vi "CODCr固定站质控流程 (子VI).vi"(9 "CODCr量程切换":enum32{"H", "L", "AUTO"}(ring)=enum."AUTO", 10 "CODCr":bool) -> (3 "布尔":bool)   [LabVIEW 2016, in "质控单元.lvlib"]
panel:
  out "参数 out":T1
  out "CODCr中断报警":bool
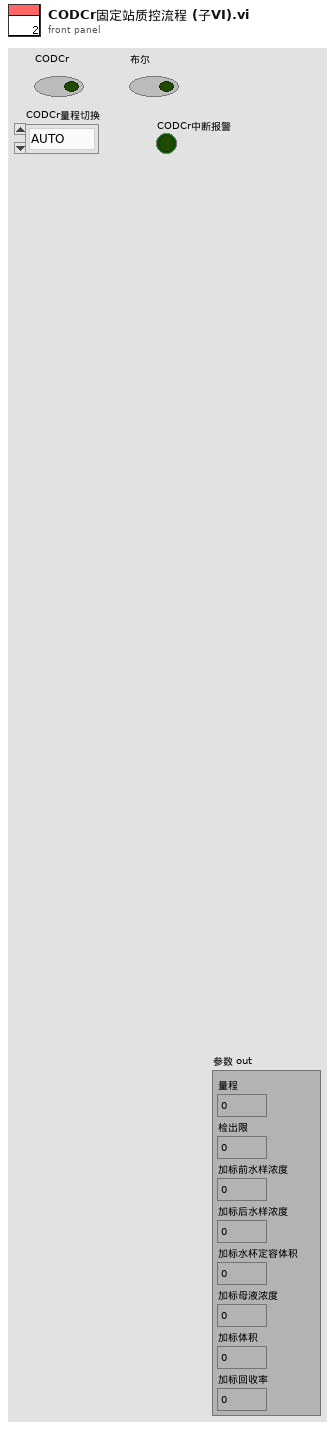
[diagram p1: front panel]
types:
  T1 = cluster{"量程":dbl, "检出限":dbl, "加标前水样浓度":dbl, "加标后水样浓度":dbl, "加标水杯定容体积":dbl, "加标母液浓度":dbl, "加标体积":dbl, "加标回收率":dbl}
  T2 = enum16{"待机", "启动水样测量", "水样测量中", "启动加标", "启动加标回收", "加标回收测量中", "结束"}
  T3 = cluster{"测量模式":enum16{"水样测量", "标样核查", "零点核查", "跨度核查", "空白测试", "加标回收", "平行样", "校零", "校标"}}
  T4 = enum16{"空闲", "水样测试", "标样核查", "零点核查", "跨度核查", "空白测试", "平行样测试", "加标回收", "空白校准", "标样校准", "初始化（清洗）"}
  T5 = cluster{"系统时间":timestamp, "工作状态":enum16{"空闲", "水样测试", "标样核查", "零点核查", "跨度核查", "空白测试", "平行样测试", "加标回收", "空白校准", "标样校准", "初始化（清洗）"}, "测量模式":enum16{"待机", "连续模式", "周期模式", "定点模式", "受控模式", "手动模式"}, "告警代码":enum16{"无告警", "缺试剂告警", "缺水样告警", "缺蒸馏水告警", "缺标液告警", "仪表漏液告警", "标定异常告警", "超量程告警", "加热异常", "低试剂预警", "超上限告警", "超下限告警", "仪表内部其他异常", "滴定异常告警", "电极异常告警", "量程切换告警", "参数设置告警", "PH电极电位异常", "电导率电极异常", "浊度光度异常", "溶解氧电极异常", "溶解氧光强异常", "温度异常告警", "PH异常告警", "溶解氧异常告警", "电导率异常告警", "浊度异常告警", "叶绿素异常告警", "藻密度异常告警", "蓝绿藻异常告警", "ORP异常告警", "氨氮异常告警", "清洁刷异常告警", "SD卡异常告警", "蓝牙异常告警", "Wifi异常告警", "流程异常告警"}, "故障代码":enum16{"无故障", "电机故障", "温度故障", "通讯故障", "滴定故障"}, "日志代码":u16, "软件版本":u16, "F0":sgl, "F1":sgl, "F2":sgl, "F3":sgl, "T":sgl, "H":sgl, "id":u16, "flowid":u16, "量程":u16, "总磷控温温度1":sgl, "营养盐控温温度2":sgl, "ADC":sgl}
  T6 = cluster{"因子编码":u32, "单位":u16, "标样参考值":sgl, "水样数据时间":timestamp, "水样实测值":sgl, "水样数据标识":string, "标样数据时间":timestamp, "标样实测值":sgl, "标样数据标识":string, "空白数据时间":timestamp, "空白实测值":sgl, "空白数据标识":string, "零点核查数据时间":timestamp, "零点核查实测值":sgl, "零点核查数据标识":string, "跨度核查数据时间":timestamp, "跨度核查实测值":sgl, "跨度核查数据标识":string, "加标回收数据时间":timestamp, "加标回收实测值":sgl, "加标回收数据标识":string, "平行样数据时间":timestamp, "平行样实测值":sgl, "平行样数据标识":string}
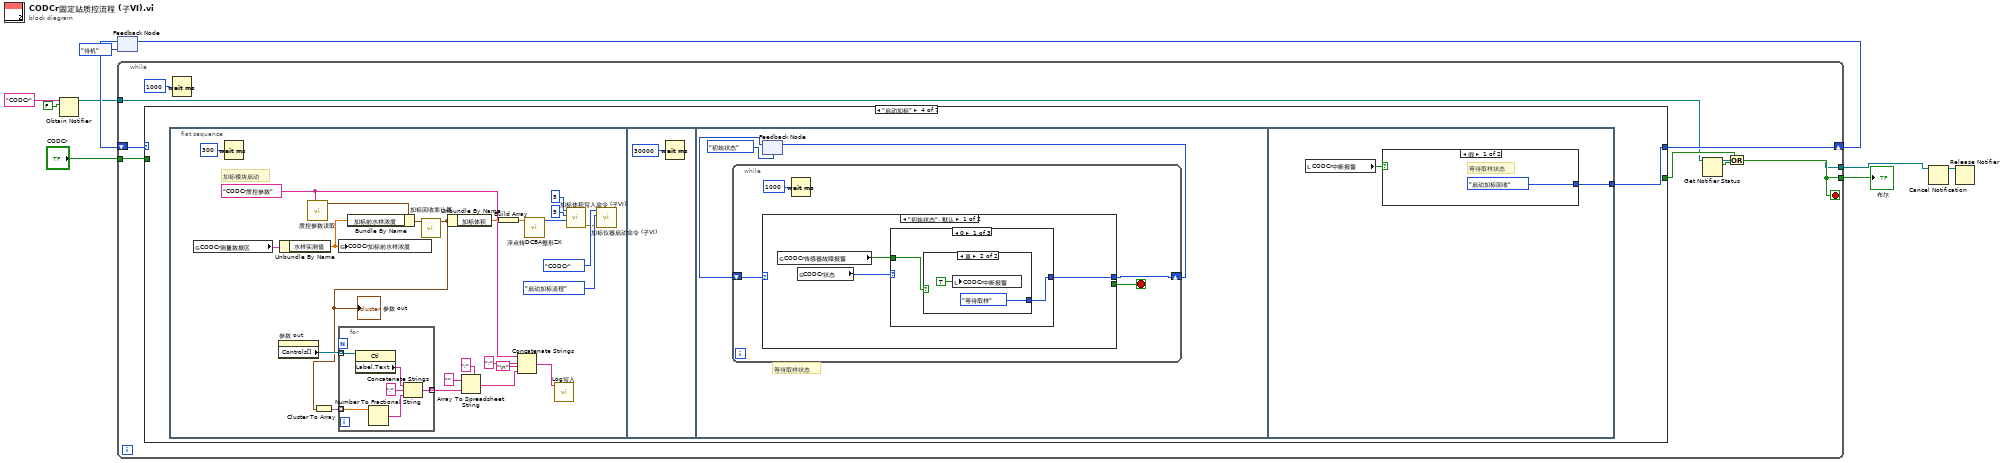
[diagram p0: block diagram]
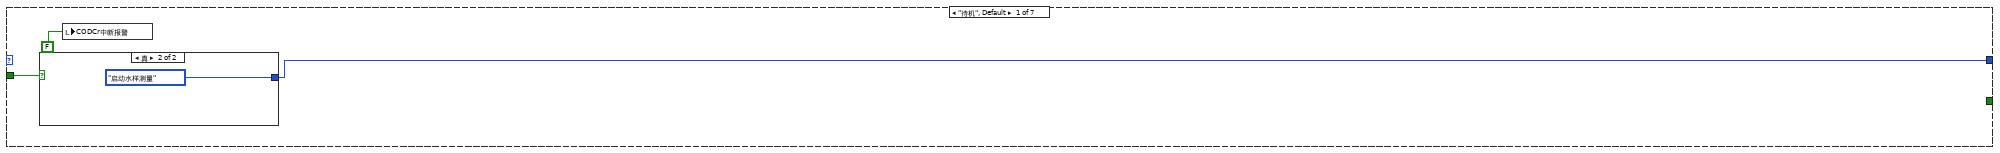
[diagram p2: hidden frame]
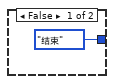
[diagram p3: hidden frame]
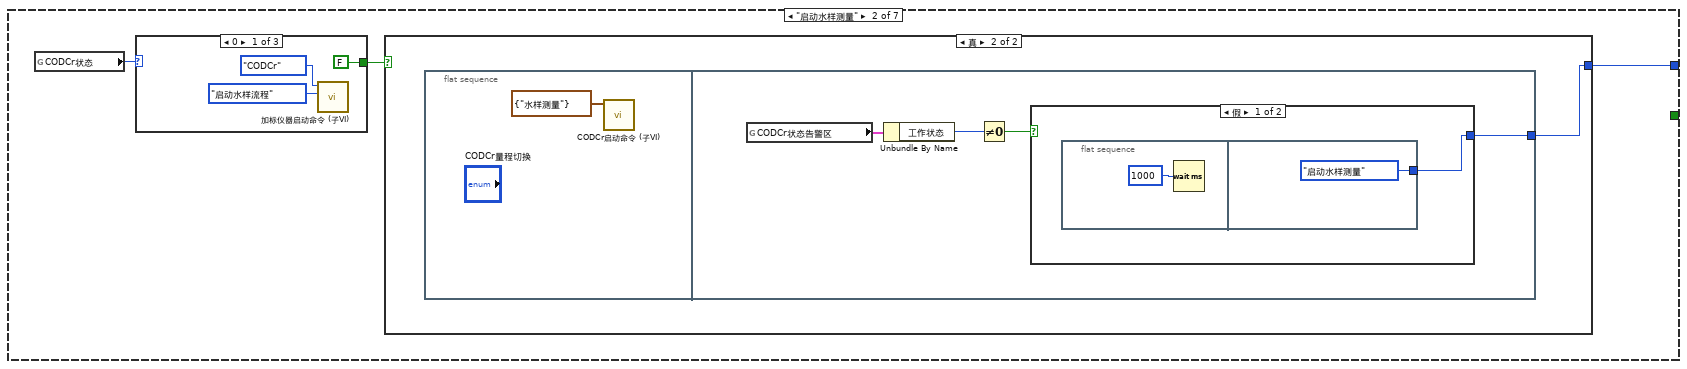
[diagram p4: hidden frame]
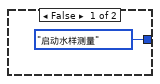
[diagram p5: hidden frame]
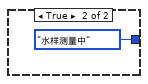
[diagram p6: hidden frame]
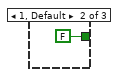
[diagram p7: hidden frame]
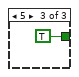
[diagram p8: hidden frame]
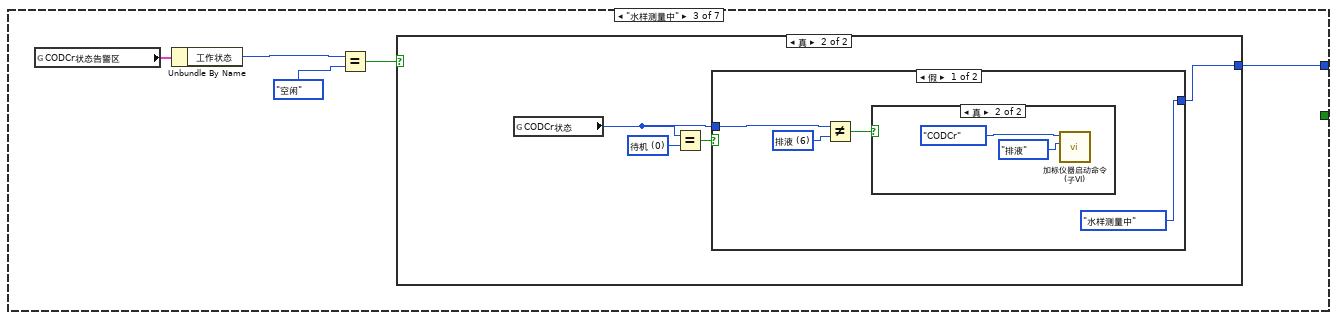
[diagram p9: hidden frame]
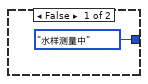
[diagram p10: hidden frame]
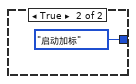
[diagram p12: hidden frame]
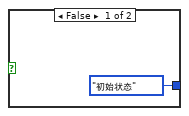
[diagram p13: hidden frame]
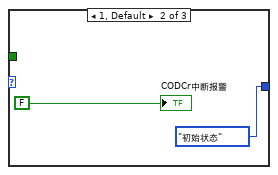
[diagram p14: hidden frame]
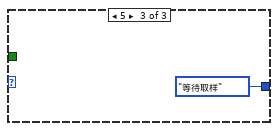
[diagram p15: hidden frame]
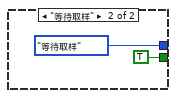
[diagram p16: hidden frame]
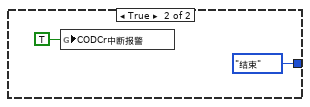
[diagram p17: hidden frame]
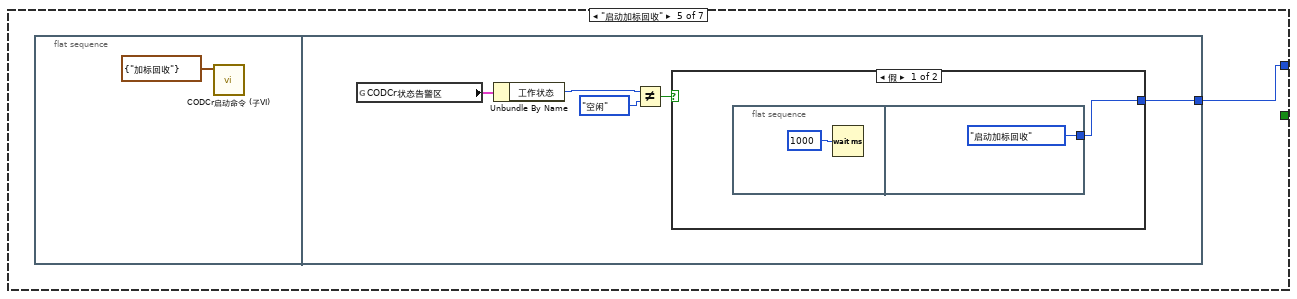
[diagram p18: hidden frame]
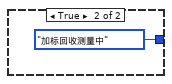
[diagram p19: hidden frame]
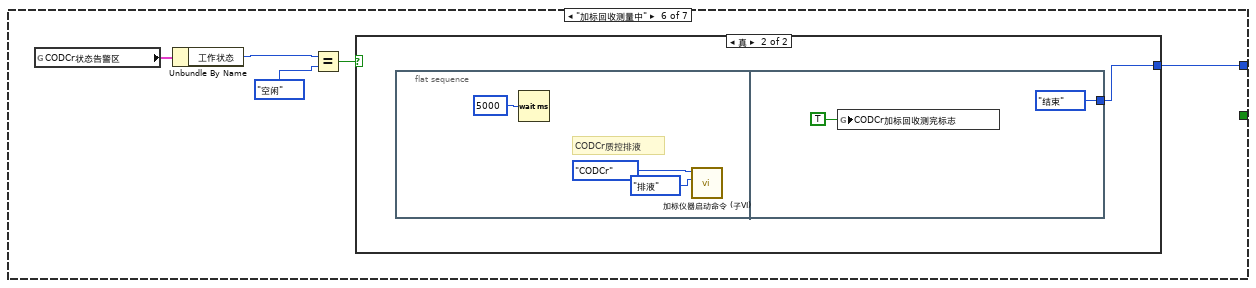
[diagram p20: hidden frame]
diagram:
  n1 = Obtain Notifier(name (unnamed)="CODCr" ("名称（未命名）"), notification data type=FALSE) -> (notifier out=w3:refnum<notifier>)  [unwired: 2 in, 2 out]
  n2 = feedback #1(T2."待机") -> (w6:T2)
  n3 = while {
    tunnel: "CODCr" -> [w19]
    tunnel: [w13] -> w8
    shift-right: [w18] -> w9
    shift-left: w6 -> [w17]
    tunnel: w3 -> [w12]
    tunnel: [w11] -> w1
    stop <- w13 stop-if-true
    n4 = case shown="\"启动加标\"" w17 {
      tunnel: [w22 w27 w48 w61 w118 w133 T2."结束"] -> w18
      tunnel: [_ _ _ _ _ _ TRUE] -> w14
      tunnel: w19 -> [w21 _ _ _ _ _ _]
      frame "待机", Default {
        n5 = case shown="真" w21 {
          tunnel: [T2."结束" T2."启动水样测量"] -> w22
          frame False {
          }
          frame True {
          }
        }
        n6 = local write "CODCr中断报警"(FALSE ("CODMn中断报警")) -> ()
      }
      frame "启动水样测量" {
        n7 = global read "加标回收状态全局变量.vi" "CODCr状态"() -> (w26:u16)
        n8 = case shown="0" w26 {
          tunnel: [FALSE ("s") FALSE ("s") TRUE ("s")] -> w25
          frame 0 {
            n9 = call "加标仪器启动命令 (子VI).vi"("启动命令"=enum16{"启动水样流程", "启动加标流程", "排液", "停止"}."启动水样流程", "仪器"=enum16{"", "氨氮", "总磷", "总氮", "CODMn", "CODCr"}."CODCr") -> ()  [unwired: 9 in, 1 out]
          }
          frame 1, Default {
          }
          frame 5 {
          }
        }
        n10 = case shown="真" w25 {
          tunnel: [T2."启动水样测量" w29] -> w27
          frame False {
          }
          frame True {
            n11 = flat-sequence {
              tunnel: [w34] -> w29
              frame #0 {
                n12 = call "CODCr启动命令 (子VI).vi"("启动测量模式"=T3 {"测量模式"=enum."水样测量"}) -> ()  [unwired: 10 in, 1 out]
              }
              frame #1 {
                n13 = global read "与CODCr交互全局.vi" "CODCr状态告警区"() -> (w32:T5)
                n14 = Unbundle By Name(w32) -> ("工作状态"=w33:T4)
                n15 = Not Equal To 0?(x=w33) -> (x != 0?=w31:bool)
                n16 = case shown="假" w31 {
                  tunnel: [w35 T2."水样测量中"] -> w34
                  frame False {
                    n17 = flat-sequence {
                      tunnel: [T2."启动水样测量"] -> w35
                      frame #0 {
                        n18 = Wait (ms)(milliseconds to wait=u32 1000 ("等待时间（毫秒）")) -> ()  [unwired: 1 out]
                      }
                      frame #1 {
                      }
                    }
                  }
                  frame True {
                  }
                }
              }
            }
          }
        }
      }
      frame "水样测量中" {
        n19 = global read "与CODCr交互全局.vi" "CODCr状态告警区"() -> (w45:T5)
        n20 = Unbundle By Name(w45) -> ("工作状态"=w44:T4)
        n21 = Equal?(x=w44, y=T4."空闲") -> (x = y?=w46:bool)
        n22 = case shown="真" w46 {
          tunnel: [T2."水样测量中" w53] -> w48
          frame False {
          }
          frame True {
            w52 = u16 0 items=["待机", "润洗", "进样", "进样完成", "柱塞泵加标", "等待取液", "排液"] ("CODCr状态")
            n23 = global read "加标回收状态全局变量.vi" "CODCr状态"() -> (w50:u16)
            n24 = Equal?(x=w50, y=w52) -> (x = y?=w51:bool)
            n25 = case shown="假" w51 {
              tunnel: [T2."水样测量中" T2."启动加标"] -> w53
              tunnel: w50 -> [w54 _]
              frame False {
                w56 = u16 6 items=["待机", "润洗", "进样", "进样完成", "柱塞泵加标", "等待取液", "排液"] ("氨氮状态")
                n26 = Not Equal?(x=w54, y=w56) -> (x != y?=w55:bool)
                n27 = case shown="真" w55 {
                  frame False {
                  }
                  frame True {
                    n28 = call "加标仪器启动命令 (子VI).vi"("启动命令"=enum16{"启动水样流程", "启动加标流程", "排液", "停止"}."排液", "仪器"=enum16{"", "氨氮", "总磷", "总氮", "CODMn", "CODCr"}."CODCr") -> ()  [unwired: 9 in, 1 out]
                  }
                }
              }
              frame True {
              }
            }
          }
        }
      }
      frame "启动加标" {
        n29 = flat-sequence {
          tunnel: [w114] -> w61
          frame #0 {
            w62 = "CODCr质控参数" ("section")
            # "加标模块启动"
            n30 = global read "与CODCr交互全局.vi" "CODCr测量数据区"() -> (w80:T6)
            n31 = Wait (ms)(milliseconds to wait=u32 300 ("等待时间（毫秒）")) -> ()  [unwired: 1 out]
            n32 = property on="参数 out" class="Clust (严格)"() -> ("Controls[]"=w68:refnum<vi>[])  [unwired: 2 in, 2 out]
            n33 = Unbundle By Name(w80) -> ("水样实测值"=w81:sgl)
            n34 = call "质控参数读取.vi"("section"=w62) -> ("参数"=w84:T1)  [unwired: 9 in, 1 out]
            n35 = global write "水样浓度全局.vi" "CODCr加标前水样浓度"(w81) -> ()
            n36 = Bundle By Name(cluster=w84, "加标前水样浓度"=w81) -> (w85:T1)
            n37 = call "加标回收率计算.vi"("参数"=w85) -> ("参数 out"=w63:T1)  [unwired: 9 in, 1 out]
            "参数 out" <- w63
            n38 = Cluster To Array(cluster=w63) -> (array=w70:dbl[])
            n39 = for {
              tunnel: w68 -> [w91] mode=indexing
              tunnel: w70 -> [w89] mode=indexing
              tunnel: [w86] -> w69 mode=indexing
              n40 = property class="Ctl"(reference=w91) -> ("Label.Text"=w90:string)  [unwired: 1 in, 2 out]
              n41 = Number To Fractional String(number=w89) -> (F-format string=w87:string)  [unwired: 3 in]
              n42 = Concatenate Strings(w90, ":" ("字符串"), w87) -> (w86:string)
            }
            n43 = Unbundle By Name(w63) -> ("加标体积"=w83:dbl)
            n44 = Array To Spreadsheet String(delimiter (Tab)=";" ("分隔符(Tab)"), array=w69, 3:"") -> (spreadsheet string=w66:string)
            n45 = Build Array(w83) -> (w79:dbl[])
            n46 = Concatenate Strings(w62, ":" ("字符串"), "\n", w66) -> (w64:string)
            n47 = call "浮点转DCBA整形ZK.vi"("浮点数"=w79) -> ("DCBA整形输出"=w74:u16[])  [unwired: 10 in]
            n48 = call "Log写入.vi"("Log"=w64) -> ()  [unwired: 11 in]
            n49 = call "加标体积写入命令 (子VI).vi"("values"=w74, "starting address"=u16 5, "Slave ID"=u16 5 ("value")) -> ("错误输出"=w73:errorcluster)  [unwired: 8 in]
            n50 = call "加标仪器启动命令 (子VI).vi"("错误输入（无错误）"=w73, "启动命令"=enum16{"启动水样流程", "启动加标流程", "排液", "停止"}."启动加标流程", "仪器"=enum16{"", "氨氮", "总磷", "总氮", "CODMn", "CODCr"}."CODCr") -> ()  [unwired: 8 in, 1 out]
          }
          frame #1 {
            n51 = Wait (ms)(milliseconds to wait=u32 30000 ("等待时间（毫秒）")) -> ()  [unwired: 1 out]
          }
          frame #2 {
            # "等待取样状态"
            n52 = feedback #2(enum16{"初始状态", "等待取样"}."初始状态") -> (w94:enum16{"初始状态", "等待取样"})
            n53 = while {
              shift-right: [w98] -> w95
              shift-left: w94 -> [w99]
              stop <- w97 stop-if-true
              n54 = case shown="\"初始状态\", 默认" w99 {
                tunnel: [w102 enum16{"初始状态", "等待取样"}."等待取样"] -> w98
                tunnel: [_ TRUE] -> w97
                frame "初始状态", Default {
                  n55 = global read "质控中断报警全局.vi" "CODCr传感器故障报警"() -> (w100:bool)
                  n56 = global read "加标回收状态全局变量.vi" "CODCr状态"() -> (w101:u16)
                  n57 = case shown="0" w101 {
                    tunnel: [w104 enum16{"初始状态", "等待取样"}."初始状态" enum16{"初始状态", "等待取样"}."等待取样"] -> w102
                    tunnel: w100 -> [w103 _ _]
                    frame 0 {
                      n58 = case shown="真" w103 {
                        tunnel: [enum16{"初始状态", "等待取样"}."初始状态" enum16{"初始状态", "等待取样"}."等待取样"] -> w104
                        frame False {
                        }
                        frame True {
                          n59 = local write "CODCr中断报警"(TRUE ("氨氮中断报警")) -> ()
                        }
                      }
                    }
                    frame 1, Default {
                      "CODCr中断报警" <- FALSE ("总氮中断报警")
                    }
                    frame 5 {
                    }
                  }
                }
                frame "等待取样" {
                }
              }
              n60 = Wait (ms)(milliseconds to wait=u32 1000 ("等待时间（毫秒）")) -> ()  [unwired: 1 out]
            }
            n61 = feedback-in #2(w95) -> ()
          }
          frame #3 {
            n62 = local read "CODCr中断报警"() -> (w113:bool)
            n63 = case shown="假" w113 {
              tunnel: [T2."启动加标回收" T2."结束"] -> w114
              frame False {
                # "等待取样状态"
              }
              frame True {
                n64 = global write "质控中断报警全局.vi" "CODCr中断报警"(TRUE ("CODCr中断报警")) -> ()
              }
            }
          }
        }
      }
      frame "启动加标回收" {
        n65 = flat-sequence {
          tunnel: [w124] -> w118
          frame #0 {
            n66 = call "CODCr启动命令 (子VI).vi"("启动测量模式"=T3 {"测量模式"=enum."加标回收"}) -> ()  [unwired: 10 in, 1 out]
          }
          frame #1 {
            n67 = global read "与CODCr交互全局.vi" "CODCr状态告警区"() -> (w123:T5)
            n68 = Unbundle By Name(w123) -> ("工作状态"=w122:T4)
            n69 = Not Equal?(x=w122, y=T4."空闲") -> (x != y?=w120:bool)
            n70 = case shown="假" w120 {
              tunnel: [w125 T2."加标回收测量中"] -> w124
              frame False {
                n71 = flat-sequence {
                  tunnel: [T2."启动加标回收"] -> w125
                  frame #0 {
                    n72 = Wait (ms)(milliseconds to wait=u32 1000 ("等待时间（毫秒）")) -> ()  [unwired: 1 out]
                  }
                  frame #1 {
                  }
                }
              }
              frame True {
              }
            }
          }
        }
      }
      frame "加标回收测量中" {
        n73 = global read "与CODCr交互全局.vi" "CODCr状态告警区"() -> (w130:T5)
        n74 = Unbundle By Name(w130) -> ("工作状态"=w129:T4)
        n75 = Equal?(x=w129, y=T4."空闲") -> (x = y?=w131:bool)
        n76 = case shown="真" w131 {
          tunnel: [T2."加标回收测量中" w135] -> w133
          frame False {
          }
          frame True {
            n77 = flat-sequence {
              tunnel: [T2."结束"] -> w135
              frame #0 {
                # "CODCr质控排液"
                n78 = Wait (ms)(milliseconds to wait=u32 5000 ("等待时间（毫秒）")) -> ()  [unwired: 1 out]
                n79 = call "加标仪器启动命令 (子VI).vi"("启动命令"=enum16{"启动水样流程", "启动加标流程", "排液", "停止"}."排液", "仪器"=enum16{"", "氨氮", "总磷", "总氮", "CODMn", "CODCr"}."CODCr") -> ()  [unwired: 9 in, 1 out]
              }
              frame #1 {
                n80 = global write "质控测完标志全局 1.vi" "CODCr加标回收测完标志"(TRUE ("COD加标回收测完标志")) -> ()
              }
            }
          }
        }
      }
      frame "结束" {
        n81 = Wait (ms)(milliseconds to wait=u32 5000 ("等待时间（毫秒）")) -> ()  [unwired: 1 out]
      }
    }
    n82 = Wait (ms)(milliseconds to wait=u32 1000 ("等待时间（毫秒）")) -> ()  [unwired: 1 out]
    n83 = Get Notifier Status(notifier=w12) -> (notifier out=w11:refnum<notifier>, current notification=w15:bool)  [unwired: 1 in, 3 out]
    n84 = Or(x=w14, y=w15) -> (x .or. y?=w13:bool)
  }
  "布尔" <- w8
  n85 = feedback-in #1(w9) -> ()
  n86 = Cancel Notification(0:w1) -> (8:w2:refnum<notifier>)  [unwired: 1 in, 2 out]
  n87 = Release Notifier(notifier=w2) -> ()  [unwired: 2 in, 3 out]
